vi "Boolean to Disable.vi"(1 "Disable?":bool) -> (0 "Disabled":T1(ring))   [LabVIEW 2023]
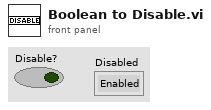
[diagram p1: front panel]
types:
  T1 = enum8{"Enabled", "Disabled", "Disabled and Grayed Out"}
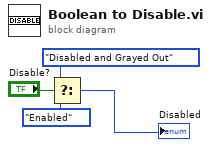
[diagram p0: block diagram]
diagram:
  n1 = Select(t=T1."Disabled and Grayed Out" ("Disabled"), s="Disable?", f=T1."Enabled" ("Disabled")) -> (s? t:f=→"Disabled":T1)
